vi "Write Ignore Mode.vi"(8 "Error In":errorcluster, 10 "Ignore Mode":T1 items=["Normal", "Merge", "Ignore"], 11 "Channel In":refnum<class "Channel.lvclass">) -> (0 "Error Out":errorcluster, 3 "Channel Out":refnum<class "Channel.lvclass">)   [LabVIEW 2018, in "Toolkit.lvlib" / "Channel.lvclass"]
uses:
  Channel.lvclass
  Typedefs/Ignore Modes.ctl
  Channel.lvclass/Channel.ctl
  Session/Session.lvclass/Session.ctl
  SSH/SSH.lvclass/SSH.ctl
  Session/Session.lvclass
  Toolkit.lvlib
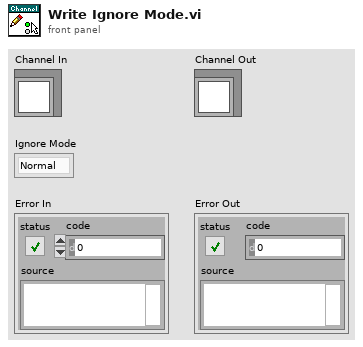
[diagram p1: front panel]
types:
  T1 = typedef "Toolkit.lvlib/Channel.lvclass/Ignore Modes.ctl" = i32
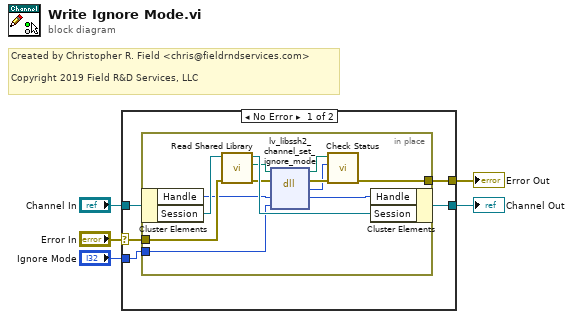
[diagram p0: block diagram]
diagram:
  # "Created by Christopher R. Field <chris@fieldrndservices.com>\n\nCopyright 2019 Field R&D Services, LLC"
  n1 = case shown="No Error" "Error In" {
    selector: "Error In" -> [w8 w24]
    tunnel: [w7 w24] -> w4
    tunnel: "Channel In" -> [w10 w23]
    tunnel: [w9 w23] -> w2
    tunnel: "Ignore Mode" -> [w6 _]
    frame No Error {
      n2 = in-place {
        in-place-border: w8 -> [w18]
        in-place-border: [w14] -> w7
        in-place-border: w6 -> [w11]
        n3 = in-place-cluster #1(w10) -> ("Handle"=w16:u64, "Session"=w22:refnum<class "Session.lvclass">)
        n4 = call "Read Shared Library.vi"("Error In"=w18, "Session In"=w22) -> ("Erorr Out"=w19:errorcluster, "libssh2lv Shared Library"=w20:path, "Session Out"=w21:refnum<class "Session.lvclass">)  [unwired: 7 in]
        n5 = dll-call lib="libssh2lv.*" fn="lv_libssh2_channel_set_ignore_mode"(path in=w20, error in=w19, "handle"=w16, "mode"=w11) -> (path out=w13:path, error out=w17:errorcluster, "status"=w12:i32, "handle"=w15:u64)  [unwired: 2 in]
        n6 = call "Check Status.vi"("Error In"=w17, "Status"=w12, "lv-libssh2 Shared Library In"=w13) -> ("Error Out"=w14:errorcluster)  [unwired: 7 in, 1 out]
        n7 = in-place-cluster #1("Handle"=w15, "Session"=w21) -> (w9:refnum<class "Channel.lvclass">)
      }
    }
    frame Error {
    }
  }
  "Error Out" <- w4
  "Channel Out" <- w2
